vi "Fit.vi"(8 "error in (no error)":errorcluster caption="entrée d'erreur (pas d'erreur)", 9 "y":string[][](array[string]), 10 "X":string[][](array[string]), 11 "OrdinalEncoder.lvclass":refnum<class "OrdinalEncoder.lvclass">) -> (0 "error out":errorcluster caption="sortie d'erreur", 2 "String Data":string, 3 "OrdinalEncoder.lvclass":refnum<class "OrdinalEncoder.lvclass">)   [LabVIEW 2020, in "OrdinalEncoder.lvclass"]
doc: "Fit the OrdinalEncoder to X.\n\nReturns : \n\n- String : OK"
uses:
  OrdinalEncoder.lvclass
  OrdinalEncoder.lvclass/OrdinalEncoder.ctl
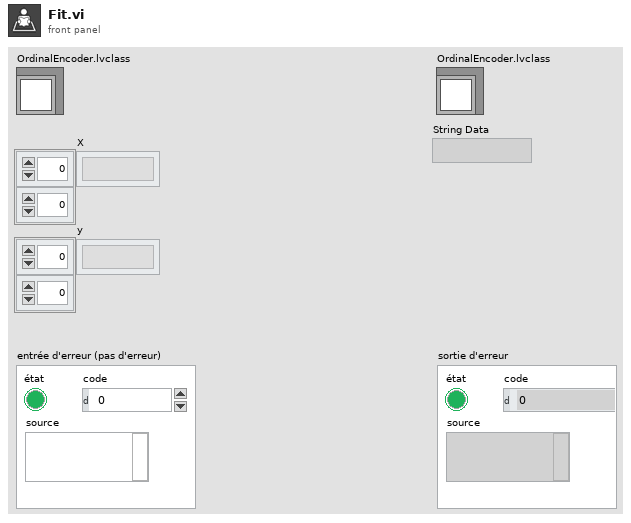
[diagram p1: front panel]
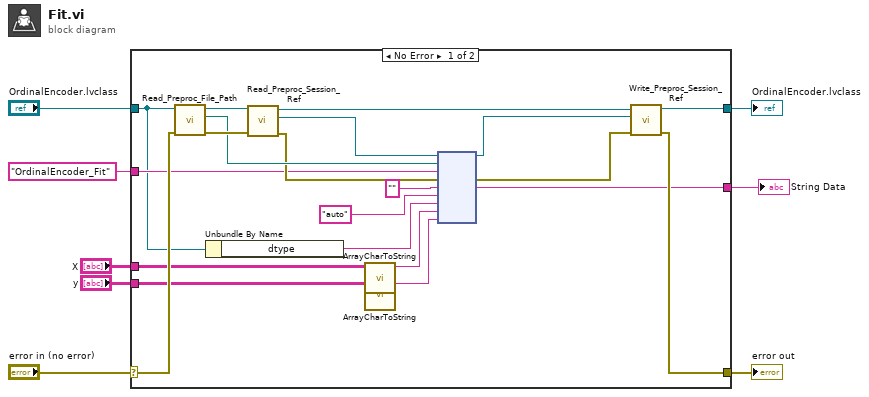
[diagram p0: block diagram]
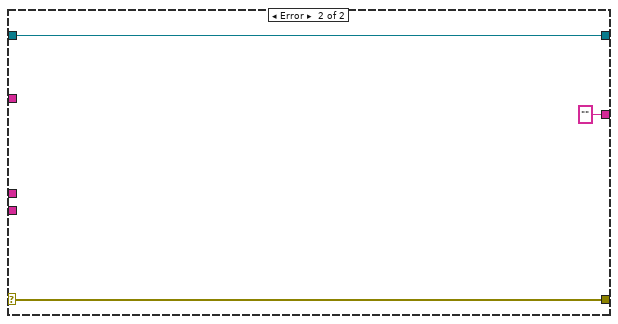
[diagram p2: hidden frame]
diagram:
  n1 = case shown="No Error" "error in (no error)" {
    selector: "error in (no error)" -> [w18 w32]
    tunnel: [w17 w32] -> w7
    tunnel: [w19 w31] -> w5
    tunnel: "OrdinalEncoder.lvclass" -> [w14 w31]
    tunnel: "OrdinalEncoder_Fit" ("Fonction") -> [w16 _]
    tunnel: [w15 ""] -> w3
    tunnel: "X" -> [w12 _]
    tunnel: "y" -> [w10 _]
    frame No Error {
      n2 = call-dynamic "Read_Preproc_File_Path.vi"("error in (no error)"=w18, "Python in"=w14) -> ("error out"=w28:errorcluster, "File_Path"=w25:path, "Python out"=w29:refnum<class "OrdinalEncoder.lvclass">)  [unwired: 7 in]
      n3 = Unbundle By Name(w14) -> ("dtype"=w20:string)
      n4 = call-dynamic "Read_Preproc_Session_Ref.vi"("error in (no error)"=w28, "Python in"=w29) -> ("error out"=w24:errorcluster, "Session_ref"=w26:refnum<k35>, "Python out"=w27:refnum<class "OrdinalEncoder.lvclass">)  [unwired: 7 in]
      n5 = call "ArrayCharToString.vi"("TAB"=w12) -> ("Instruction"=w11:string)  [unwired: 10 in]
      n6 = call "ArrayCharToString.vi"("TAB"=w10) -> ("Instruction"=w9:string)  [unwired: 10 in]
      n7 = node(w26, w25, w16, w24, "", "auto", w20, w11, w9) -> (w22:refnum<k35>, w23:errorcluster, w15:string)  [unwired: 4 in, 2 out]
      n8 = call-dynamic "Write_Preproc_Session_Ref.vi"("error in (no error)"=w23, "Session_ref"=w22, "Python in"=w27) -> ("error out"=w17:errorcluster, "Python out"=w19:refnum<class "OrdinalEncoder.lvclass">)  [unwired: 7 in]
    }
    frame Error {
    }
  }
  "error out" <- w7
  "OrdinalEncoder.lvclass" <- w5
  "String Data" <- w3
